vi "car_Error_main.vi"(7 "Command (Check for Error)":T3=enum."Check for Error", 8 "error in (no error)":errorcluster, 10 "Error User Event":T2, 11 "Consumer Queue Refnum":T1) -> (0 "error out":errorcluster)   [LabVIEW 2009]
doc: "This VI is the main VI for the error module. This VI will shutdown the application cleanly if an error occurs.\n\nThe errors can then be reported back."
uses:
  car_Error_Command_enum.ctl
  controls/car_ErrorUserEvent_refnum.ctl
  controls/car_ConsumerQueue_refnum.ctl
  controls/car_ConsumerDataType_cluster.ctl
  controls/car_ConsumerCommand_enum.ctl
panel:
  # "Inputs"
  # "Outputs"
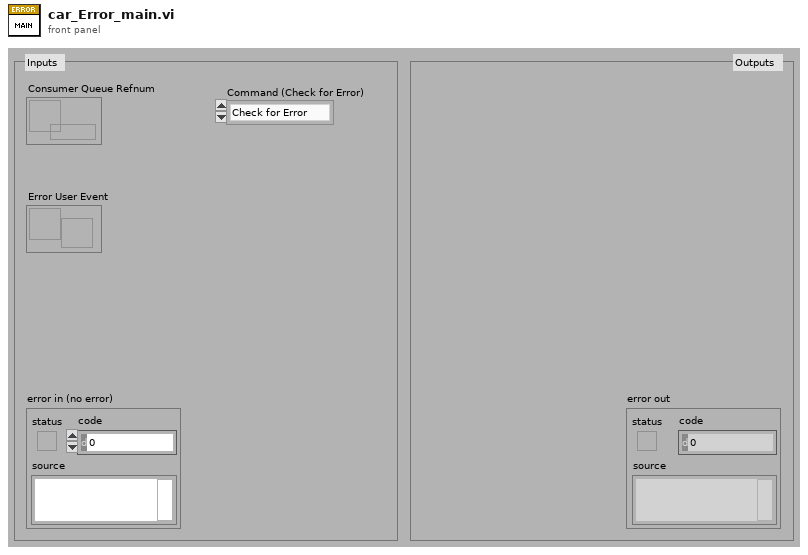
[diagram p1: front panel]
types:
  T1 = typedef "car_ConsumerQueue_refnum.ctl" = refnum<queue>
  T2 = typedef "car_ErrorUserEvent_refnum.ctl" = refnum<user-event>
  T3 = typedef "car_Error_Command_enum.ctl" = enum16{"Initialise", "Check for Error", "Report Errors"}
  T4 = typedef "car_ConsumerDataType_cluster.ctl" = cluster{"Command":T5, "Data":variant}
  T5 = typedef "car_ConsumerCommand_enum.ctl" = enum16{"Initialise", "Update Start Car Wash Display", "Start Wash", "Check Car Wash", "Car Wash Completed", "Exit"}
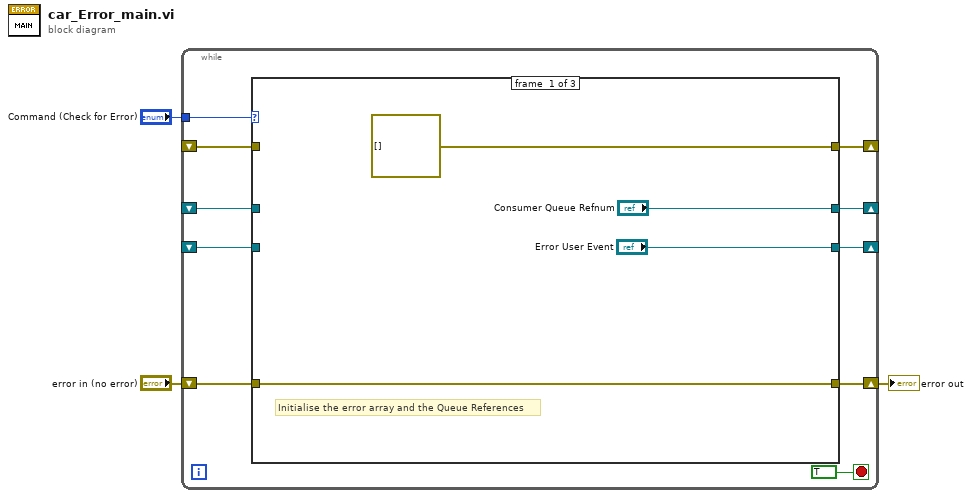
[diagram p0: block diagram]
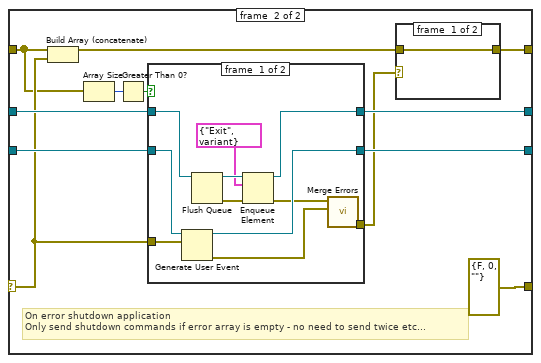
[diagram p3: hidden frame]
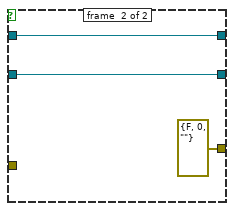
[diagram p4: hidden frame]
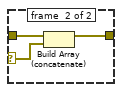
[diagram p5: hidden frame]
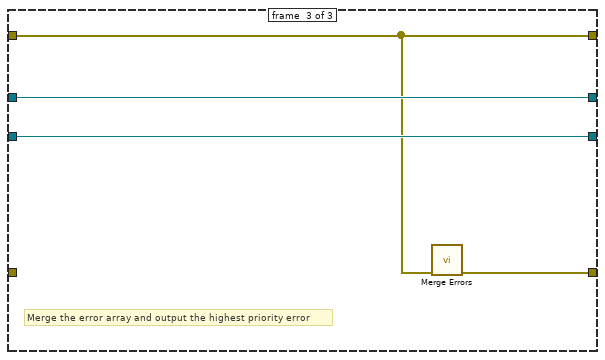
[diagram p6: hidden frame]
diagram:
  n1 = while {
    shift-right: [w12] -> w2
    shift-left: "error in (no error)" -> [w13]
    tunnel: "Command (Check for Error)" -> [w10]
    shift-right: [w9] -> _
    shift-left: _ -> [w7]
    shift-right: [w8] -> _
    shift-left: _ -> [w6]
    shift-right: [w5] -> _
    shift-left: _ -> [w4]
    stop <- TRUE stop-if-true
    n2 = case shown="\"Check for Error\"" w10 {
      tunnel: w13 -> [w17 w25 _]
      tunnel: [w17 w24 w60] -> w12
      tunnel: ["Consumer Queue Refnum" w21 w63] -> w9
      tunnel: ["Error User Event" w20 w62] -> w8
      tunnel: w7 -> [_ w23 w63]
      tunnel: w6 -> [_ w22 w62]
      tunnel: [errorcluster[] [] w18 w61] -> w5
      tunnel: w4 -> [_ w19 w61]
      frame #0 {
        # "Initialise the error array and the Queue References"
      }
      frame #1 {
        n3 = case shown="Error" w25 {
          selector: w25 -> [w29 w37]
          tunnel: [w29 errorcluster {"status"=FALSE, "code"=0, "source"=""} ("error IO")] -> w24
          tunnel: w23 -> [w28 w41]
          tunnel: w22 -> [w27 w39]
          tunnel: [w28 w40] -> w21
          tunnel: [w27 w38] -> w20
          tunnel: w19 -> [w26 w32]
          tunnel: [w26 w34] -> w18
          frame #0 {
            # "No error - do nothing"
          }
          frame #1 {
            # "On error shutdown application\nOnly send shutdown commands if error array is empty - no need to send twice etc..."
            n4 = Build Array (concatenate)(w32, w37) -> (w33:errorcluster[])
            n5 = Array Size(array=w32) -> (size(s)=w31:i32)
            n6 = Greater Than 0?(x=w31) -> (x > 0?=w30:bool)
            n7 = case shown="False" w30 {
              tunnel: w41 -> [w51 w55]
              tunnel: [w50 w55] -> w40
              tunnel: w39 -> [w48 w54]
              tunnel: [w47 w54] -> w38
              tunnel: w37 -> [w44 _]
              tunnel: [w43 errorcluster {"status"=FALSE, "code"=0, "source"=""} ("error out")] -> w35
              frame #0 {
                n8 = Generate User Event(user event=w48, event data cluster=w44) -> (user event out=w47:T2, error out=w45:errorcluster)  [unwired: 1 in]
                n9 = Flush Queue(queue=w51) -> (queue out=w52:T1, error out=w49:errorcluster)  [unwired: 1 in, 1 out]
                n10 = Enqueue Element(queue=w52, element=T4 {"Command"=enum."Exit", "Data"=variant}, error in (no error)=w49) -> (queue out=w50:T1, error out=w46:errorcluster)  [unwired: 1 in, 1 out]
                n11 = call <vilib>:"Merge Errors.vi"("error in 2 (no error)"=w45, "error in 1 (no error)"=w46) -> ("error out"=w43:errorcluster)  [unwired: 5 in]
              }
              frame #1 {
              }
            }
            n12 = case shown="Error" w35 {
              selector: w35 -> [_ w57]
              tunnel: w33 -> [w56 w59]
              tunnel: [w56 w58] -> w34
              frame #0 {
              }
              frame #1 {
                n13 = Build Array (concatenate)(w59, w57) -> (w58:errorcluster[])
              }
            }
          }
        }
      }
      frame #2 {
        # "Merge the error array and output the highest priority error"
        n14 = call <vilib>:"Merge Errors.vi"("error array in"=w61) -> ("error out"=w60:errorcluster)  [unwired: 6 in]
      }
    }
  }
  "error out" <- w2
